vi "main.vi"() -> ()   [LabVIEW 2024]
uses:
  Controls/#typedef_program_data_soundDB.ctl
  <vilib>/Utility/miscctls.llb/LVPoint32TypeDef.ctl
  Controls/#typedef_program_states_soundDB.ctl
panel:
  out "Program States":T1
  out "error out":errorcluster
  in  "error in (no error)":errorcluster
  in  "Cluster":T2={"Sound intensity [dB]"=0, "Sound intensity: MIN"=0.0, "Sound intensity: MAX"=230.0, "Char array"=[], "Point32"={"Horizontal"=0, "Vertical"=0}, "drag?"=FALSE, "offset"={"Horizontal"=0, "Vertical"=0}} {"Sound intensity [dB]" scale=0.0..100.0}
  out "Limit exceeded?":bool
  in  "Stop Button":bool
  out "To be moved":string
  in  "Sound intensity: MAX":dbl=230.0
  in  "Sound intensity: MIN":dbl
  in  "Sound intensity [dB]":u8(slide) scale=0.0..100.0
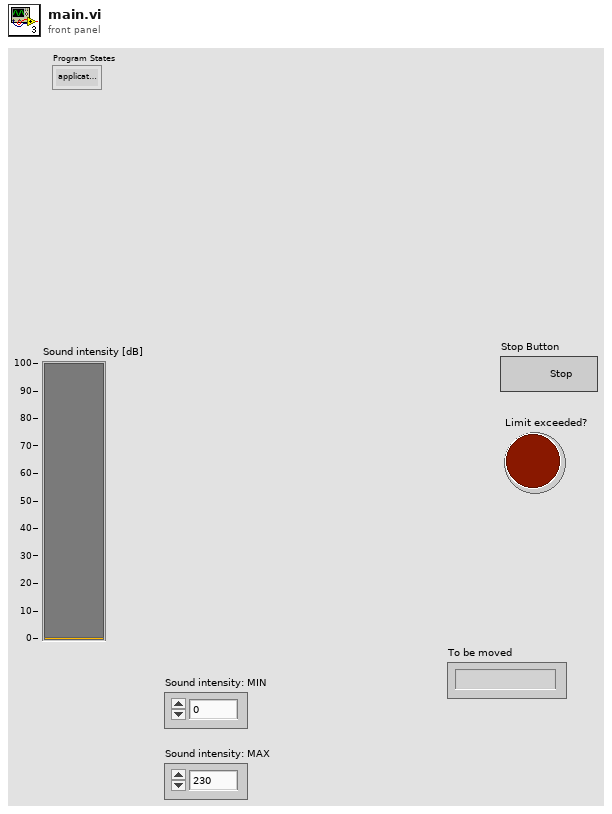
[diagram p1: front panel]
types:
  T1 = typedef "#typedef_program_states_soundDB.ctl" = enum16{"application error", "init", "idle", "move", "Limit exceeded", "exit"}
  T2 = typedef "#typedef_program_data_soundDB.ctl" = cluster{"Sound intensity [dB]":u8, "Sound intensity: MIN":dbl, "Sound intensity: MAX":dbl, "Char array":i16[], "Point32":T3, "drag?":bool, "offset":T3}
  T3 = typedef "LVPoint32TypeDef.ctl" = cluster{"Horizontal":i32, "Vertical":i32}
  T4 = typedef "LVPositionTypeDef.ctl" = cluster{"Left":i32, "Top":i32}
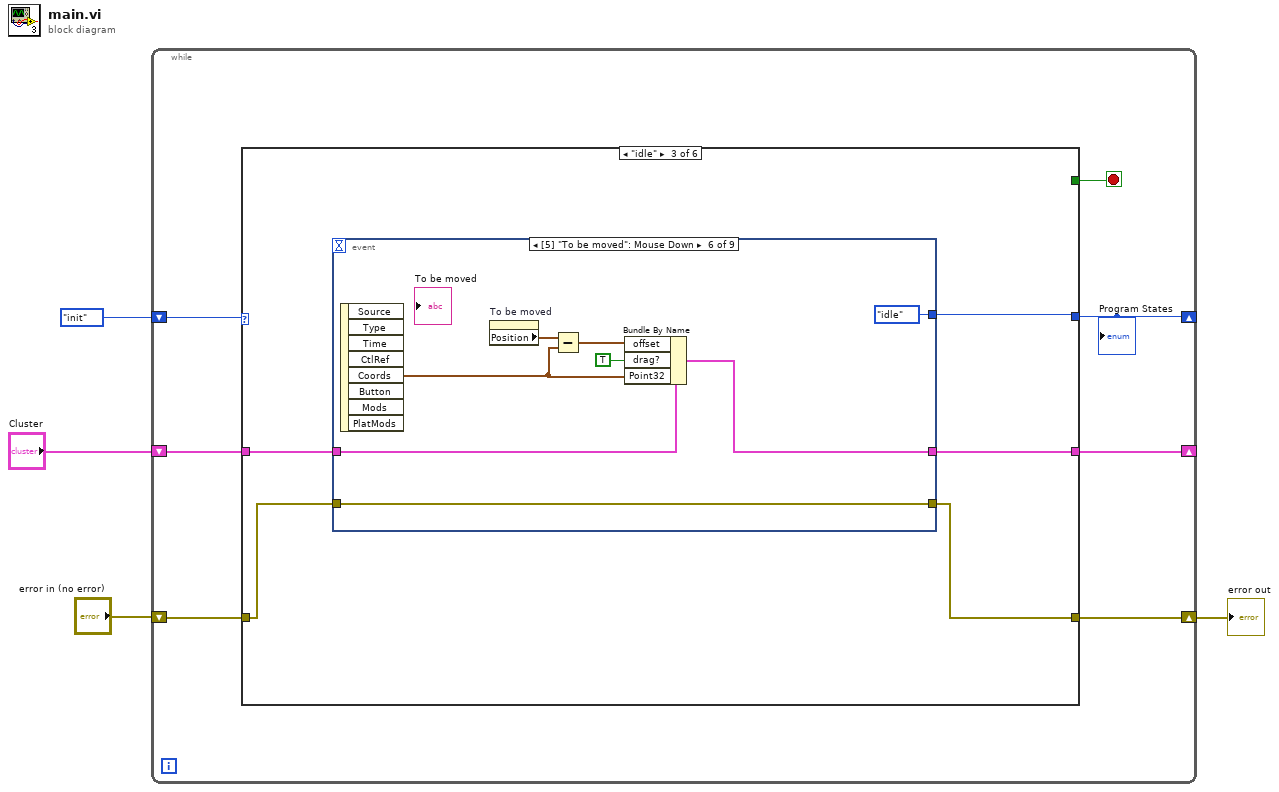
[diagram p0: block diagram]
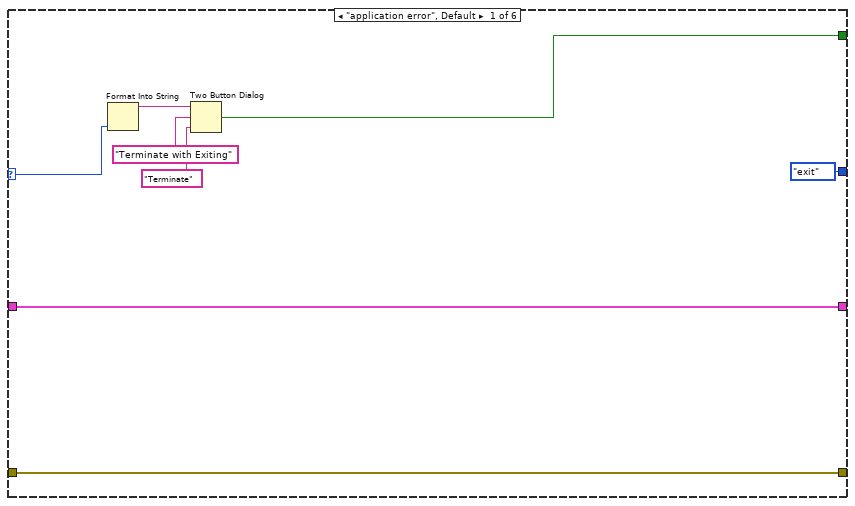
[diagram p2: hidden frame]
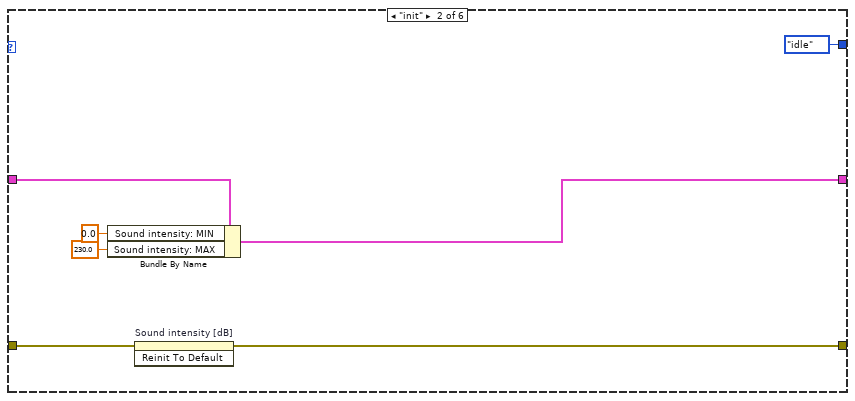
[diagram p3: hidden frame]
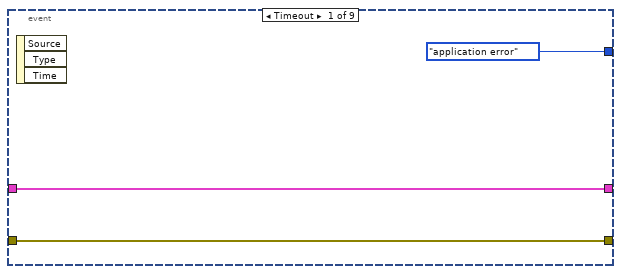
[diagram p4: hidden frame]
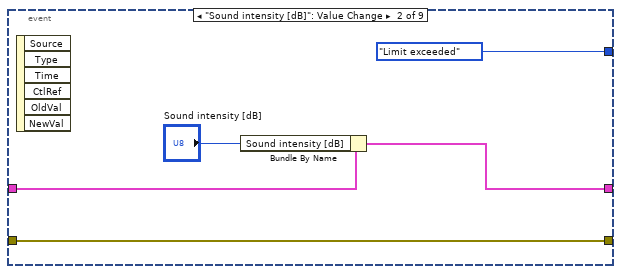
[diagram p5: hidden frame]
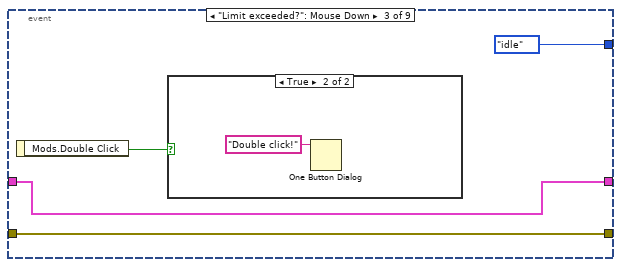
[diagram p6: hidden frame]
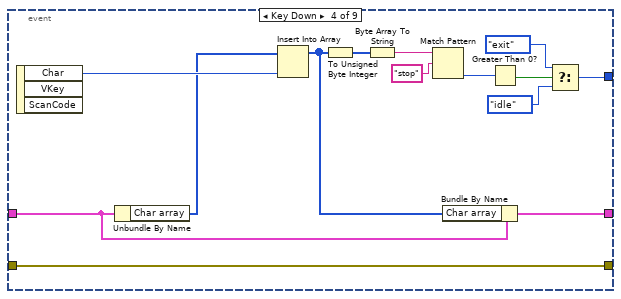
[diagram p8: hidden frame]
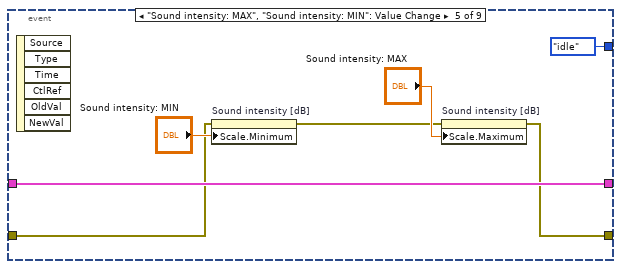
[diagram p9: hidden frame]
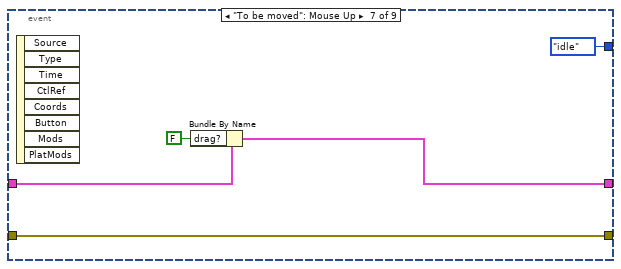
[diagram p10: hidden frame]
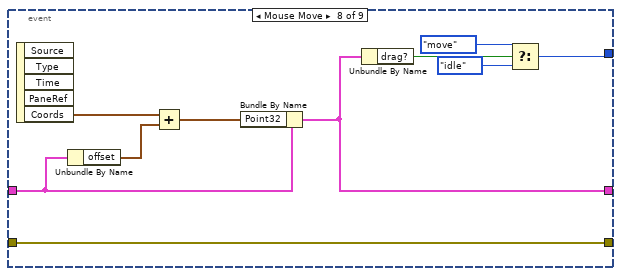
[diagram p11: hidden frame]
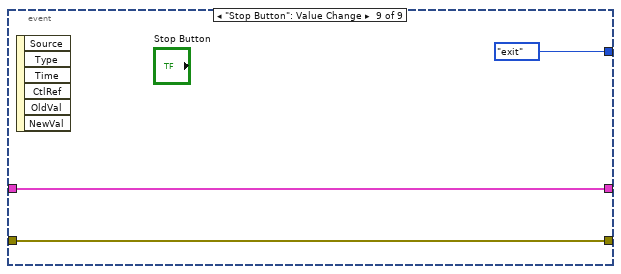
[diagram p12: hidden frame]
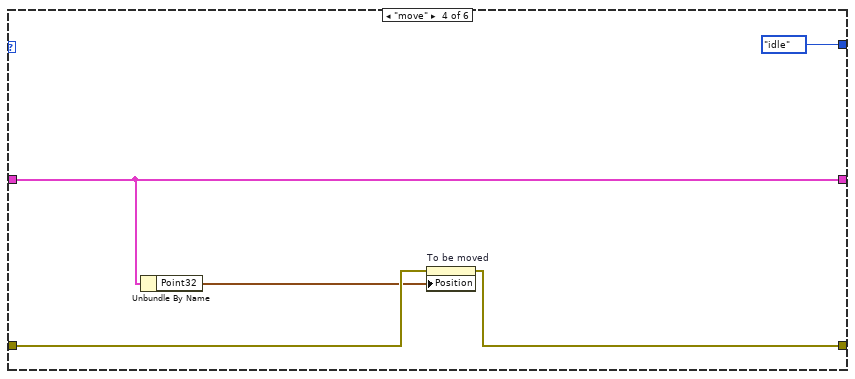
[diagram p13: hidden frame]
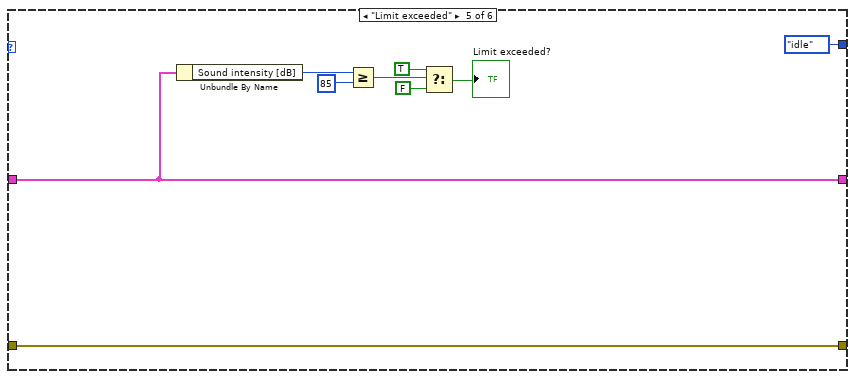
[diagram p14: hidden frame]
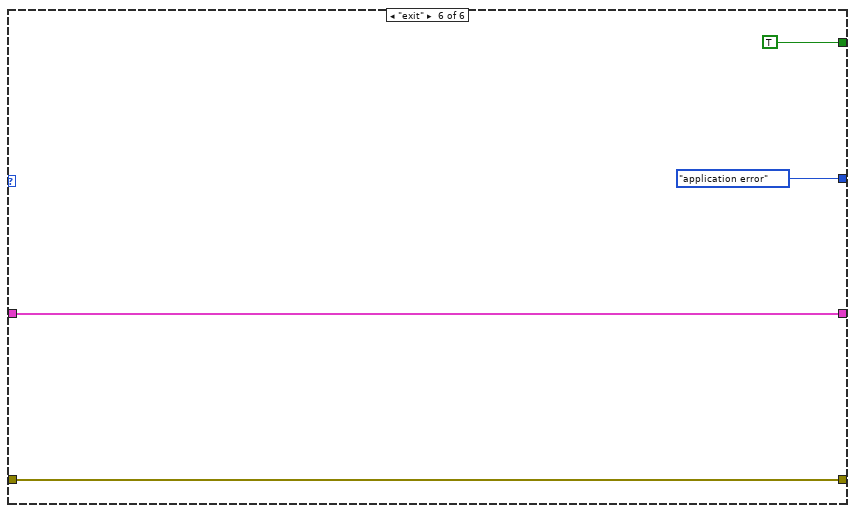
[diagram p15: hidden frame]
diagram:
  n1 = while {
    shift-right: [w9] -> _
    shift-left: #typedef_program_states_soundDB."init" ("Program States") -> [w11]
    shift-right: [w5] -> _
    shift-left: "Cluster" -> [w8]
    shift-right: [w6] -> w1
    shift-left: "error in (no error)" -> [w7]
    stop <- w10 stop-if-true
    n2 = case shown="\"idle\"" w11 {
      selector: w11 -> [w19 _ _ _ _ _]
      tunnel: [w15 _ _ _ _ TRUE] -> w10
      tunnel: [#typedef_program_states_soundDB."exit" ("Program States") #typedef_program_states_soundDB."idle" ("Program States") w31 #typedef_program_states_soundDB."idle" ("Program States") #typedef_program_states_soundDB."idle" ("Program States") #typedef_program_states_soundDB."application error" ("Program States")] -> w9
      tunnel: w8 -> [w13 w25 w30 w96 w99 w107]
      tunnel: [w13 w22 w29 w96 w99 w107] -> w5
      tunnel: w7 -> [w12 w21 w28 w94 w97 w106]
      tunnel: [w12 w20 w27 w93 w97 w106] -> w6
      frame "application error", Default {
        n3 = Format Into String(w19) -> (resulting string=w18:string)  [unwired: 3 in, 1 out]
        n4 = Two Button Dialog(message=w18, 1:"Terminate" ("F button name (\"Cancel\")"), 2:"Terminate with Exiting" ("T button name (\"OK\")")) -> (T button?=w15:bool)
      }
      frame "init" {
        n5 = Bundle By Name(cluster=w25, "Sound intensity: MIN"=0.0, "Sound intensity: MAX"=230.0) -> (w22:T2)
        n6 = invoke on="Sound intensity [dB]" class="Slide (strict)" method="Reinit To Default"(error in=w21) -> (error out=w20:errorcluster)  [unwired: 2 in, 2 out]
      }
      frame "idle" {
        n7 = event shown="[5] \"To be moved\": Mouse Down" {
          selector: _ -> [_ _ _ _ _ _ _ _ _]
          dyn-events: _ -> [_ _ _ _ _ _ _ _ _]
          timeout: _ -> [_ _ _ _ _ _ _ _ _]
          tunnel: [#typedef_program_states_soundDB."application error" ("Program States") #typedef_program_states_soundDB."Limit exceeded" ("Program States") #typedef_program_states_soundDB."idle" ("Program States") w47 #typedef_program_states_soundDB."idle" ("Program States") #typedef_program_states_soundDB."idle" ("Program States") #typedef_program_states_soundDB."idle" ("Program States") w85 #typedef_program_states_soundDB."exit" ("Program States")] -> w31
          tunnel: w30 -> [w33 w37 w41 w56 w62 w67 w78 w80 w90]
          tunnel: [w33 w36 w41 w57 w62 w66 w76 w84 w90] -> w29
          tunnel: w28 -> [w32 w35 w40 w45 w61 w71 w74 w83 w89]
          tunnel: [w32 w35 w40 w45 w59 w71 w74 w83 w89] -> w27
          event Timeout {
            n8 = event-data() -> ()  [unwired: 1 in, 3 out]
          }
          event "Sound intensity [dB]": Value Change {
            n9 = event-data() -> ()  [unwired: 1 in, 6 out]
            n10 = Bundle By Name(cluster=w37, "Sound intensity [dB]"="Sound intensity [dB]") -> (w36:T2)
          }
          event "Limit exceeded?": Mouse Down {
            n11 = event-data() -> ("Mods.Double Click"=w43:bool)  [unwired: 1 in]
            n12 = case shown="True" w43 {
              frame False {
              }
              frame True {
                n13 = One Button Dialog(message="Double click!") -> ()  [unwired: 1 in, 1 out]
              }
            }
          }
          event Key Down {
            n14 = event-data() -> ("Char"=w58:i16)  [unwired: 1 in, 2 out]
            n15 = Unbundle By Name(w56) -> ("Char array"=w55:i16[])
            n16 = Insert Into Array(array=w55, new element=w58) -> (w53:i16[])  [unwired: 1 in]
            n17 = To Unsigned Byte Integer(number=w53) -> (unsigned 8bit integer=w54:u8[])
            n18 = Byte Array To String(unsigned byte array=w54) -> (string=w52:string)
            n19 = Match Pattern(string=w52, regular expression="stop") -> (offset past match=w50:i32)  [unwired: 1 in, 3 out]
            n20 = Bundle By Name(cluster=w56, "Char array"=w53) -> (w57:T2)
            n21 = Greater Than 0?(x=w50) -> (x > 0?=w49:bool)
            n22 = Select(t=#typedef_program_states_soundDB."exit" ("Program States"), s=w49, f=#typedef_program_states_soundDB."idle") -> (s? t:f=w47:T1)
          }
          event "Sound intensity: MAX", "Sound intensity: MIN": Value Change {
            n23 = event-data() -> ()  [unwired: 1 in, 6 out]
            n24 = property on="Sound intensity [dB]" class="Slide (strict)"(error in=w61, "Scale.Minimum"="Sound intensity: MIN") -> (error out=w60:errorcluster)  [unwired: 1 in, 1 out]
            n25 = property on="Sound intensity [dB]" class="Slide (strict)"(error in=w60, "Scale.Maximum"="Sound intensity: MAX") -> (error out=w59:errorcluster)  [unwired: 1 in, 1 out]
          }
          event "To be moved": Mouse Down {
            n26 = event-data() -> ("Coords"=w69:T3)  [unwired: 1 in, 7 out]
            n27 = property on="To be moved" class="Str"() -> ("Position"=w70:T4)  [unwired: 2 in, 2 out]
            n28 = Subtract(x=w70, y=w69) -> (x-y=w68:T4)
            n29 = Bundle By Name(cluster=w67, "offset"=w68, "drag?"=TRUE, "Point32"=w69) -> (w66:T2)
          }
          event "To be moved": Mouse Up {
            n30 = event-data() -> ()  [unwired: 1 in, 8 out]
            n31 = Bundle By Name(cluster=w78, "drag?"=FALSE) -> (w76:T2)
          }
          event Mouse Move {
            n32 = event-data() -> ("Coords"=w82:T3)  [unwired: 1 in, 4 out]
            n33 = Unbundle By Name(w80) -> ("offset"=w79:T3)
            n34 = Add(x=w82, y=w79) -> (x+y=w81:T3)
            n35 = Bundle By Name(cluster=w80, "Point32"=w81) -> (w84:T2)
            n36 = Unbundle By Name(w84) -> ("drag?"=w88:bool)
            n37 = Select(t=#typedef_program_states_soundDB."move" ("Program States"), s=w88, f=#typedef_program_states_soundDB."idle" ("Program States")) -> (s? t:f=w85:T1)
          }
          event "Stop Button": Value Change {
            n38 = event-data() -> ()  [unwired: 1 in, 6 out]
          }
        }
      }
      frame "move" {
        n39 = Unbundle By Name(w96) -> ("Point32"=w92:T3)
        n40 = property on="To be moved" class="Str"(error in=w94, "Position"=w92) -> (error out=w93:errorcluster)  [unwired: 1 in, 1 out]
      }
      frame "Limit exceeded" {
        n41 = Unbundle By Name(w99) -> ("Sound intensity [dB]"=w98:u8)
        n42 = Greater Or Equal?(x=w98, y=u8 85) -> (x >= y?=w105:bool)
        n43 = Select(t=TRUE, s=w105, f=FALSE) -> (s? t:f=→"Limit exceeded?":bool)
      }
      frame "exit" {
      }
    }
    "Program States" <- w9
  }
  "error out" <- w1
